vi "etlOpen.vi"(1 "lens":enum16{"0", "1"}(ring)) -> ()   [LabVIEW 2017]
uses:
  <vilib>/DAQmx/write.llb/DAQmx Write (Analog 1D DBL NChan 1Samp).vi
  globalDevices.vi
  <vilib>/DAQmx/create/channels.llb/DAQmx Create Channel (AO-Voltage-Basic).vi
  globalUtilities.vi
  <vilib>/DAQmx/configure/timing.llb/DAQmx Timing (Sample Clock).vi
  <vilib>/DAQmx/miscellaneous.llb/DAQmx Fill In Error Info.vi
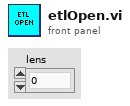
[diagram p1: front panel]
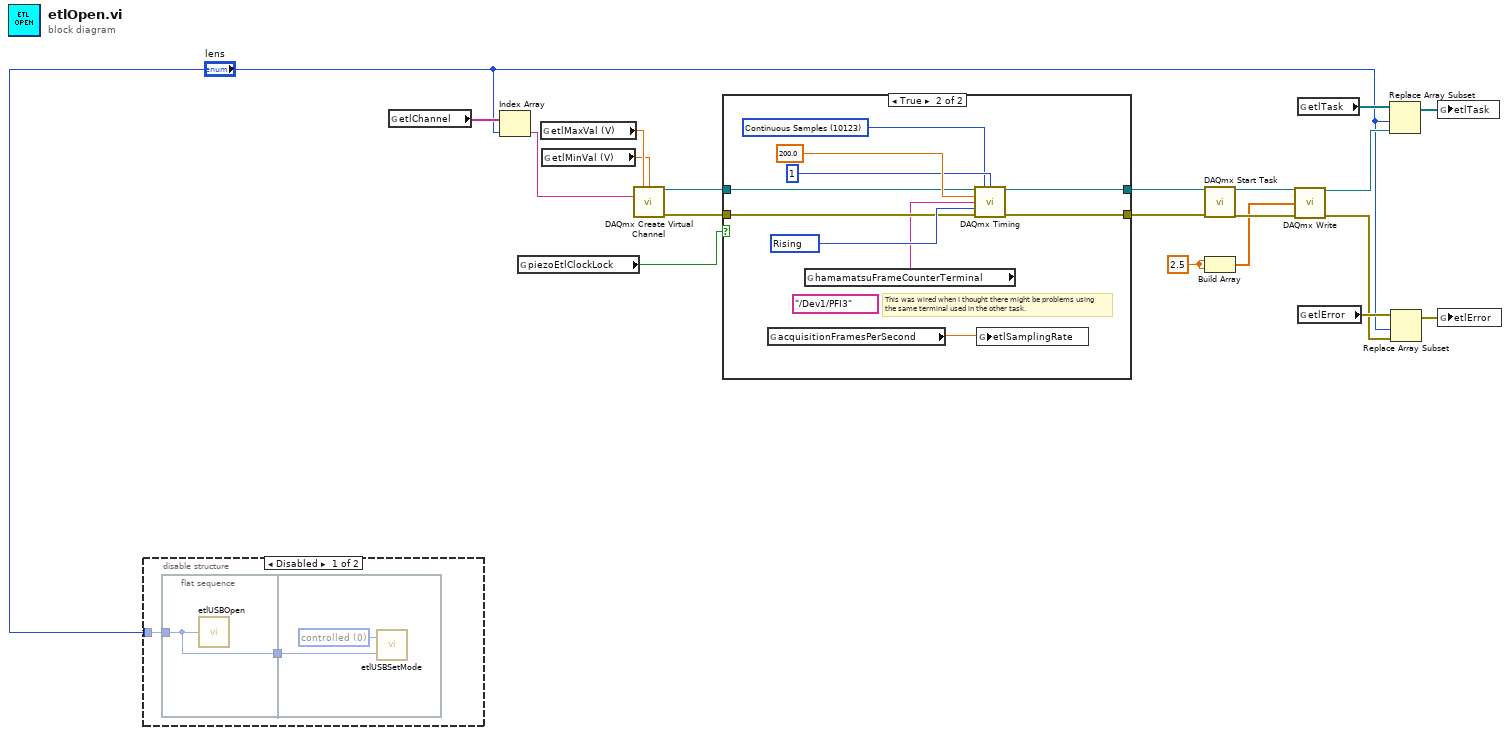
[diagram p0: block diagram]
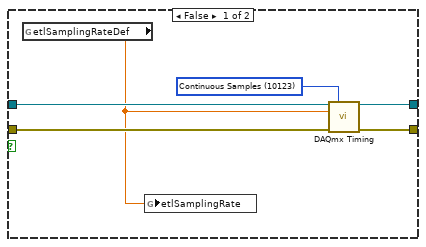
[diagram p2: hidden frame]
diagram:
  w9 = 2.5 ("data")
  n1 = disable-structure shown="Disabled" {
    disable-tunnel: "lens" -> [w21 _]
    frame Disabled {
      n2 = flat-sequence {
        tunnel: w21 -> [w23]
        tunnel: [w23] -> w22
        tunnel: w22 -> [w25]
        frame #0 {
          n3 = call "etlUSBOpen.vi"("lens"=w23) -> ()  [unwired: 1 in, 1 out]
        }
        frame #1 {
          w24 = u16 0 items=["controlled"] ("mode")
          n4 = call "etlUSBSetMode.vi"("lens"=w25, "mode"=w24) -> ()  [unwired: 1 in]
        }
      }
    }
    frame Enabled {
    }
  }
  n5 = global read "globalDevices.vi" "etlChannel"() -> (w20:tag[])
  n6 = Index Array(array=w20, index="lens") -> (element=w19:tag)
  n7 = global read "globalUtilities.vi" "piezoEtlClockLock"() -> (w1:bool)
  n8 = global read "globalDevices.vi" "etlMaxVal (V)"() -> (w7:dbl)
  n9 = global read "globalDevices.vi" "etlMinVal (V)"() -> (w6:dbl)
  n10 = call-poly <vilib>:"DAQmx Create Virtual Channel.vi"("maximum value"=w7, "minimum value"=w6, "physical channels"=w19) -> ("task out"=w5:refnum<k21>, "error out"=w4:errorcluster)  [unwired: 11 in]
  n11 = case shown="True" w1 {
    tunnel: w5 -> [w30 w37]
    tunnel: w4 -> [w29 w36]
    tunnel: [w28 w35] -> w3
    tunnel: [w27 w34] -> w2
    frame False {
      w31 = 10123 items=["Finite Samples"=10178, "Continuous Samples"=10123, "Hardware Timed Single Point"=12522] ("sample mode")
      n12 = global read "globalDevices.vi" "etlSamplingRateDef"() -> (w26:dbl)
      n13 = global write "globalDevices.vi" "etlSamplingRate"(w26) -> ()
      n14 = call-poly <vilib>:"DAQmx Timing.vi"("task/channels in"=w30, "sample mode"=w31, "rate"=w26, "error in"=w29) -> ("task out"=w28:refnum<k21>, "error out"=w27:errorcluster)  [unwired: 10 in]
    }
    frame True {
      (unwired) tag "/Dev1/PFI3" ("source")
      w41 = 10280 items=["Rising"=10280, "Falling"=10171] ("active edge")
      w38 = 10123 items=["Finite Samples"=10178, "Continuous Samples"=10123, "Hardware Timed Single Point"=12522] ("sample mode")
      # "This was wired when I thought there might be problems using \nthe same terminal used in the other task."
      n15 = global read "globalUtilities.vi" "acquisitionFramesPerSecond"() -> (w33:dbl)
      n16 = global read "globalDevices.vi" "hamamatsuFrameCounterTerminal"() -> (w32:tag)
      n17 = call-poly <vilib>:"DAQmx Timing.vi"("task/channels in"=w37, "sample mode"=w38, "samples per channel"=1, "rate"=200.0, "source"=w32, "active edge"=w41, "error in"=w36) -> ("task out"=w35:refnum<k21>, "error out"=w34:errorcluster)  [unwired: 7 in]
      n18 = global write "globalDevices.vi" "etlSamplingRate"(w33) -> ()
    }
  }
  n19 = call <vilib>:"DAQmx Start Task.vi"("task/channels in"=w3, "error in"=w2) -> ("task out"=w16:refnum<k21>, "error out"=w15:errorcluster)  [unwired: 12 in]
  n20 = Build Array(w9, w9) -> (w8:dbl[])
  n21 = call-poly <vilib>:"DAQmx Write.vi"("task/channels in"=w16, "data"=w8, "error in"=w15) -> ("task out"=w14:refnum<k21>, "error out"=w11:errorcluster)  [unwired: 10 in, 1 out]
  n22 = global read "globalDevices.vi" "etlTask"() -> (w18:refnum<k21>[])
  n23 = global read "globalDevices.vi" "etlError"() -> (w12:errorcluster[])
  n24 = Replace Array Subset(array=w18, new element=w14, index="lens") -> (w17:refnum<k21>[])
  n25 = Replace Array Subset(array=w12, new element=w11, index="lens") -> (w13:errorcluster[])
  n26 = global write "globalDevices.vi" "etlTask"(w17) -> ()
  n27 = global write "globalDevices.vi" "etlError"(w13) -> ()
